vi "Save To Clip Board.vi"(8 "error in (no error)":errorcluster, 11 "palette":string) -> (0 "error out":errorcluster, 2 "function return":u32, 3 "palette out":string)   [LabVIEW 2014, in "atmcd32d.lvlib"]
doc: "unsigned int WINAPI SaveToClipBoard(char * palette);"
uses:
  atmcd32d.lvlib
  atmcd32d.dll
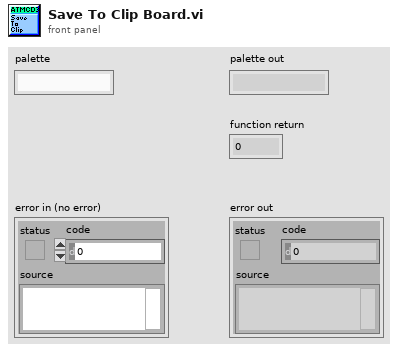
[diagram p1: front panel]
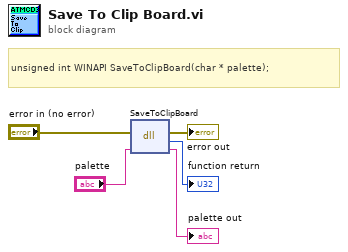
[diagram p0: block diagram]
diagram:
  # "unsigned int WINAPI SaveToClipBoard(char * palette);"
  n1 = dll-call lib="C:/Users/Bakir/Documents/Lambda2-Testing/lib/Andorlib/atmcd32d.*" fn="SaveToClipBoard"(error in="error in (no error)", "palette"="palette") -> (error out=→"error out":errorcluster, →"function return":u32, "palette"=→"palette out":string)  [unwired: 2 in, 1 out]
